vi "Close.vi"(8 "error in (no error)":errorcluster, 11 "BS120x In":refnum<class "BS120x.lvclass">) -> (0 "error out":errorcluster, 3 "BS120x Out":refnum<class "BS120x.lvclass">)   [LabVIEW 2021, in "BS120x Driver.lvlib" / "BS120x.lvclass"]
doc: "Closes the connection to the specified Battery Simulator 1200.\n(c) 2019 Bloomy Controls, Inc. All rights reserved."
uses:
  BS120x.lvclass
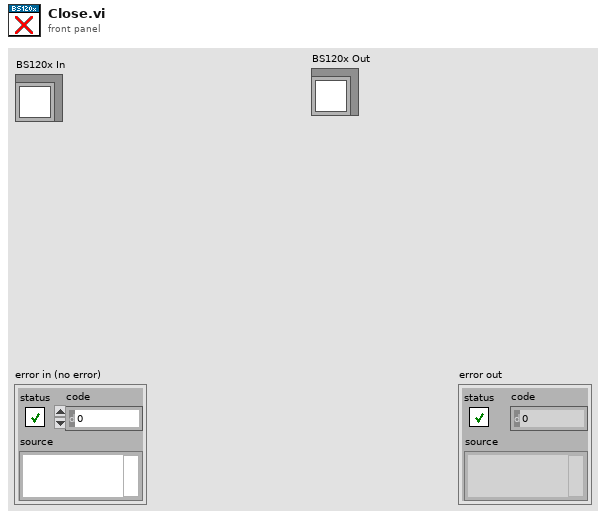
[diagram p1: front panel]
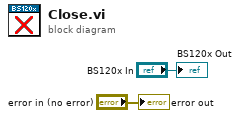
[diagram p0: block diagram]
diagram:
  "error out" <- "error in (no error)"
  "BS120x Out" <- "BS120x In"
